vi "Get Optimiser Strategy.vi"(8 "error in (no error)":errorcluster, 11 "Optimiser SBlock in":refnum<class "Optimiser SBlock.lvclass">) -> (0 "error out":errorcluster, 1 "Value":dbl, 2 "Optimisation Strategy":T1, 3 "Optimiser SBlock out":refnum<class "Optimiser SBlock.lvclass">)   [LabVIEW 2020, in "Run Utilities.lvlib" / "Optimiser SBlock.lvclass"]
uses:
  Optimiser SBlock.lvclass
  Optimiser Cell/Optimisation Strategy.ctl
  Optimiser Cell/Optimiser Cell.lvclass
  Optimiser SBlock.lvclass/Optimiser SBlock.ctl
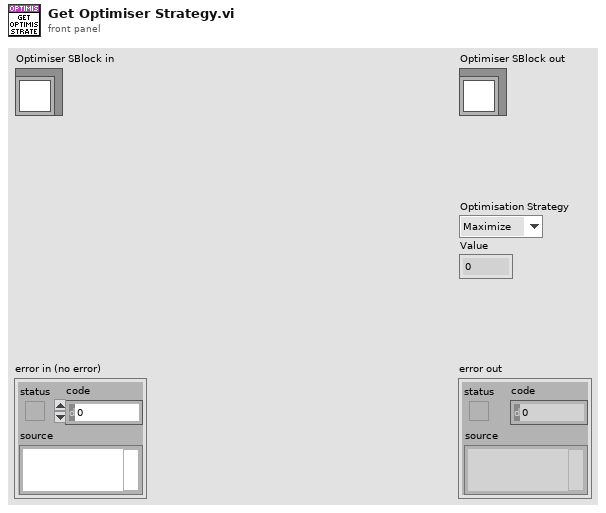
[diagram p1: front panel]
types:
  T1 = typedef "Run Utilities.lvlib/Optimiser Cell.lvclass/Optimisation Strategy.ctl" = enum16{"Maximize", "Minimize", "Value"}
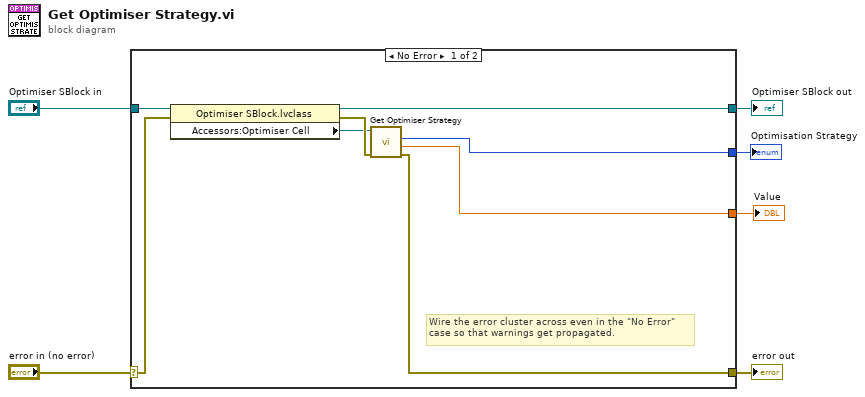
[diagram p0: block diagram]
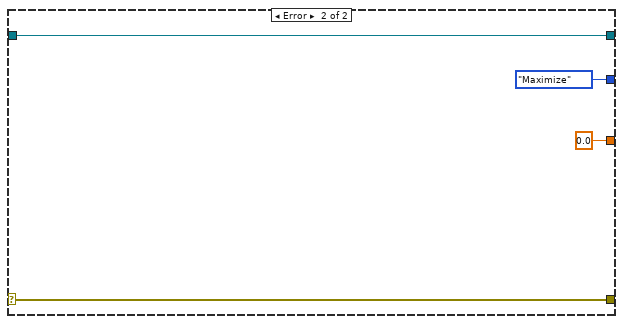
[diagram p2: hidden frame]
diagram:
  n1 = case shown="No Error" "error in (no error)" {
    selector: "error in (no error)" -> [w11 w18]
    tunnel: [w7 w18] -> w5
    tunnel: [w12 w17] -> w3
    tunnel: "Optimiser SBlock in" -> [w13 w17]
    tunnel: [w9 Optimisation_Strategy."Maximize" ("Optimisation Strategy")] -> w2
    tunnel: [w8 0.0 ("Value")] -> w1
    frame No Error {
      # "Wire the error cluster across even in the \"No Error\"\ncase so that warnings get propagated."
      n2 = property class="Optimiser SBlock.lvclass"(reference=w13, error in=w11) -> (reference out=w12:refnum<class "Optimiser SBlock.lvclass">, error out=w14:errorcluster, "Accessors:Optimiser Cell"=w10:refnum<class "Optimiser Cell.lvclass">)
      n3 = call-dynamic "Get Optimiser Strategy.vi"("error in (no error)"=w14, "Optimiser Cell in"=w10) -> ("error out"=w7:errorcluster, "Value"=w8:dbl, "Optimisation Strategy"=w9:T1)  [unwired: 6 in, 1 out]
    }
    frame Error {
    }
  }
  "error out" <- w5
  "Optimiser SBlock out" <- w3
  "Optimisation Strategy" <- w2
  "Value" <- w1
